vi "ImageProcessing_Blurr.vi"(11 "Path":path) -> (3 "2D Picture":picture)   [LabVIEW 2020]
uses:
  <vilib>/Analysis/2dsp.llb/2D Convolution (DBL).vi
  <vilib>/Analysis/NI_AALPro.lvlib
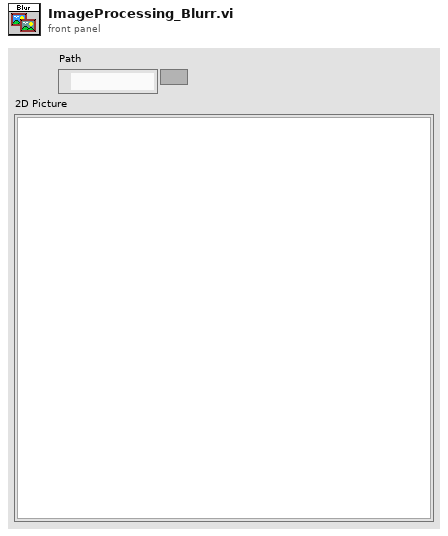
[diagram p1: front panel]
types:
  T1 = typedef "imagedata.ctl" = cluster{"image type":i32, "image depth":i32, "image":u8[], "mask":u8[], "colors":u32[], "Rectangle":cluster{"left":i16, "top":i16, "right":i16, "bottom":i16}}
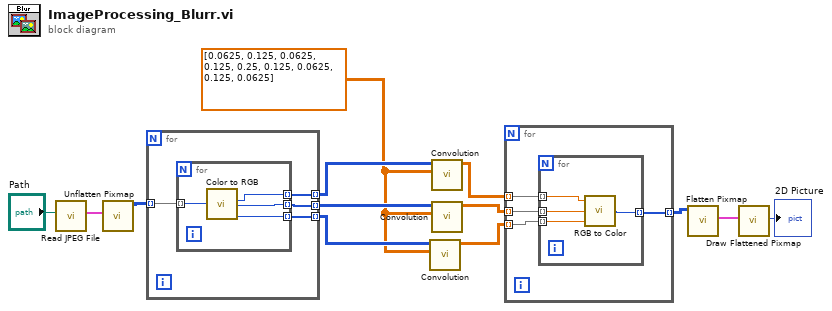
[diagram p0: block diagram]
diagram:
  w4 = dbl[][] [[0.0625, 0.125, 0.0625], [0.125, 0.25, 0.125], [0.0625, 0.125, 0.0625]]
  n1 = call <vilib>:"Read JPEG File.vi"("path to JPEG file"="Path") -> ("image data"=w12:T1)  [unwired: 8 in, 2 out]
  n2 = call <vilib>:"Unflatten Pixmap.vi"("image data"=w12) -> ("24-bit pixmap"=w11:u32[][])  [unwired: 4 in, 6 out]
  n3 = for {
    tunnel: w11 -> [w17] mode=indexing
    tunnel: [w16] -> w5 mode=indexing
    tunnel: [w15] -> w6 mode=indexing
    tunnel: [w14] -> w7 mode=indexing
    n4 = for {
      tunnel: w17 -> [w21] mode=indexing
      tunnel: [w20] -> w16 mode=indexing
      tunnel: [w19] -> w15 mode=indexing
      tunnel: [w18] -> w14 mode=indexing
      n5 = call <vilib>:"Color to RGB.vi"("Color"=w21) -> ("R"=w18:u8, "G"=w19:u8, "B"=w20:u8)  [unwired: 1 out]
    }
  }
  n6 = call-poly <vilib>:"Convolution.vi"("Y"=w4, "X"=w5) -> ("X * Y"=w1:dbl[][])  [unwired: 8 in, 1 out]
  n7 = call-poly <vilib>:"Convolution.vi"("Y"=w4, "X"=w7) -> ("X * Y"=w3:dbl[][])  [unwired: 8 in, 1 out]
  n8 = call-poly <vilib>:"Convolution.vi"("Y"=w4, "X"=w6) -> ("X * Y"=w2:dbl[][])  [unwired: 8 in, 1 out]
  n9 = for {
    tunnel: [w25] -> w8 mode=indexing
    tunnel: w3 -> [w24] mode=indexing
    tunnel: w2 -> [w23] mode=indexing
    tunnel: w1 -> [w22] mode=indexing
    n10 = for {
      tunnel: [w29] -> w25 mode=indexing
      tunnel: w24 -> [w28] mode=indexing
      tunnel: w23 -> [w27] mode=indexing
      tunnel: w22 -> [w26] mode=indexing
      n11 = call <vilib>:"RGB to Color.vi"("B"=w26, "G"=w27, "R"=w28) -> ("Color"=w29:u32)
    }
  }
  n12 = call <vilib>:"Flatten Pixmap.vi"("24-bit pixmap"=w8) -> ("image data"=w10:T1)  [unwired: 10 in]
  n13 = call <vilib>:"Draw Flattened Pixmap.vi"("image data"=w10) -> ("new picture"=→"2D Picture":picture)  [unwired: 8 in]
